vi "Double Motor Init.vi"(0 "Motor In":T2={"Motor1"={"DeviceStatus"={"status"=FALSE, "code"=0, "source"=""}, "Type"=enum."PWM", "PWM"={"PWM Channel"=enum."Invalid", "DeadBand"={"Name"="", "maxPositivePwm"=0, "minPositivePwm"=0, "centerPwm"=0, "maxNegativePwm"=0, "minNegativePwm"=0, "angularRange"=0}}, "CAN"={"Device Number"=0, "Control Mode"=enum."Percent VBus", "Semaphore"=refnum, "Max Vout"=12.0, "TalonSRX Control Mode"=enum."Percent VBus"}, "Invert"=FALSE}, "Motor2"={"DeviceStatus"={"status"=FALSE, "code"=0, "source"=""}, "Type"=enum."PWM", "PWM"={"PWM Channel"=enum."Invalid", "DeadBand"={"Name"="", "maxPositivePwm"=0, "minPositivePwm"=0, "centerPwm"=0, "maxNegativePwm"=0, "minNegativePwm"=0, "angularRange"=0}}, "CAN"={"Device Number"=0, "Control Mode"=enum."Percent VBus", "Semaphore"=refnum, "Max Vout"=12.0, "TalonSRX Control Mode"=enum."Percent VBus"}, "Invert"=FALSE}, "Last Motor Power"=0.0}, 1 "PWM Channel":T1, 5 "CAN Id":u8, 7 "Use Can":bool, 9 "Invert (default false)":bool, 11 "error in":errorcluster, 12 "PWM Channel 2":T1) -> (4 "Motor Out":T2={"Motor1"={"DeviceStatus"={"status"=FALSE, "code"=0, "source"=""}, "Type"=enum."PWM", "PWM"={"PWM Channel"=enum."Invalid", "DeadBand"={"Name"="", "maxPositivePwm"=0, "minPositivePwm"=0, "centerPwm"=0, "maxNegativePwm"=0, "minNegativePwm"=0, "angularRange"=0}}, "CAN"={"Device Number"=0, "Control Mode"=enum."Percent VBus", "Semaphore"=refnum, "Max Vout"=12.0, "TalonSRX Control Mode"=enum."Percent VBus"}, "Invert"=FALSE}, "Motor2"={"DeviceStatus"={"status"=FALSE, "code"=0, "source"=""}, "Type"=enum."PWM", "PWM"={"PWM Channel"=enum."Invalid", "DeadBand"={"Name"="", "maxPositivePwm"=0, "minPositivePwm"=0, "centerPwm"=0, "maxNegativePwm"=0, "minNegativePwm"=0, "angularRange"=0}}, "CAN"={"Device Number"=0, "Control Mode"=enum."Percent VBus", "Semaphore"=refnum, "Max Vout"=12.0, "TalonSRX Control Mode"=enum."Percent VBus"}, "Invert"=FALSE}, "Last Motor Power"=0.0}, 15 "error out":errorcluster)   [LabVIEW 2015]
uses:
  2 Motor Typedef.ctl
  <vilib>/Rock Robotics/WPI/MotorControl/WPI_MotorControlDeviceRef.ctl
  <vilib>/Rock Robotics/WPI/MotorControl/WPI_MotorControlType.ctl
  <vilib>/Rock Robotics/SystemInterfaces/DIO/FPGA_DIOPWMChannel.ctl
  <vilib>/Rock Robotics/WPI/PWM/WPI_PWMDeadband.ctl
  <vilib>/Rock Robotics/WPI/CAN/Jaguar/SubVIs/WPI_CANJaguar_ControlMode.ctl
  <vilib>/Rock Robotics/WPI/CAN/TalonSRX/WPI_CANTalonSRX_APIControlMode.ctl
  <vilib>/Rock Robotics/WPI/MotorControl/WPI_MotorControlOpenCANTalonSRX.vi
  <vilib>/Rock Robotics/WPI/MotorControl/WPI_MotorControlOpen VictorSP.vi
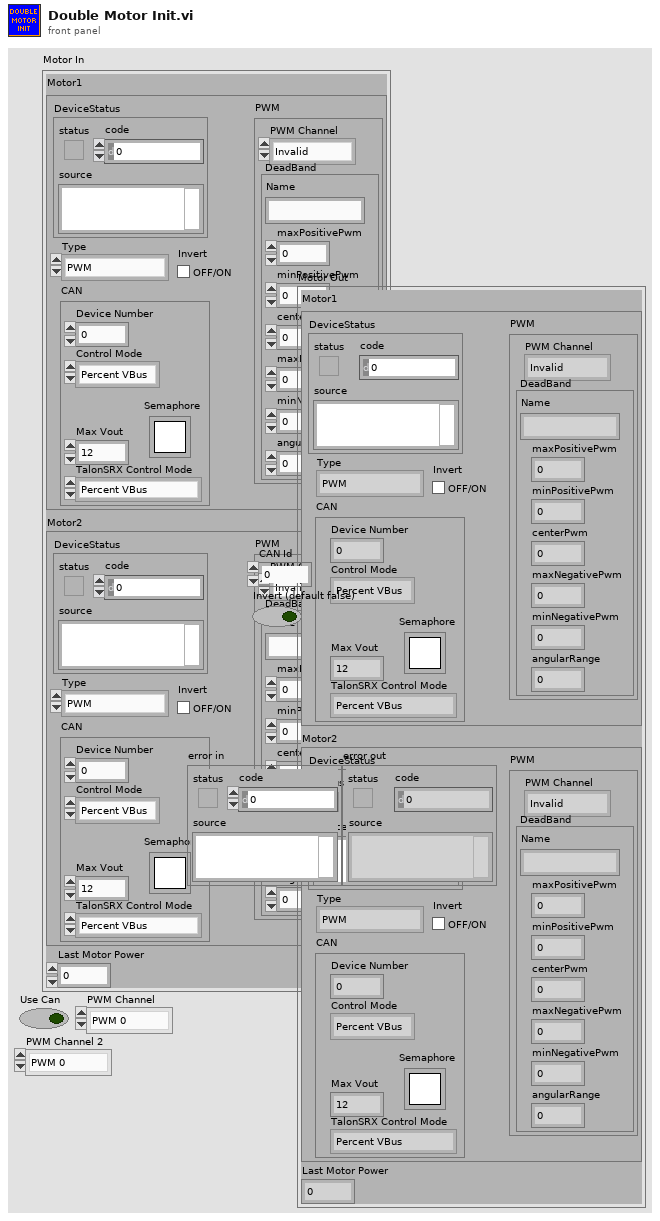
[diagram p1: front panel]
types:
  T1 = typedef "FPGA_DIOPWMChannel.ctl" = enum8{"PWM 0", "PWM 1", "PWM 2", "PWM 3", "PWM 4", "PWM 5", "PWM 6", "PWM 7", "PWM 8", "PWM 9", "PWM MXP 0", "PWM MXP 1", "PWM MXP 2", "PWM MXP 3", "PWM MXP 4", "PWM MXP 5", "PWM MXP 6", "PWM MXP 7", "PWM MXP 8", "PWM MXP 9", "Invalid"}
  T2 = typedef "2 Motor Typedef.ctl" = cluster{"Motor1":T3, "Motor2":T3, "Last Motor Power":dbl}
  T3 = typedef "WPI_MotorControlDeviceRef.ctl" = cluster{"DeviceStatus":errorcluster, "Type":T4, "PWM":cluster{"PWM Channel":T1, "DeadBand":T5}, "CAN":cluster{"Device Number":u8, "Control Mode":T6, "Semaphore":T7, "Max Vout":dbl, "TalonSRX Control Mode":T8}, "Invert":bool}
  T4 = typedef "WPI_MotorControlType.ctl" = enum16{"PWM", "CAN", "CANTalonSRX"}
  T5 = typedef "WPI_PWMDeadband.ctl" = cluster{"Name":string, "maxPositivePwm":i32, "minPositivePwm":i32, "centerPwm":i32, "maxNegativePwm":i32, "minNegativePwm":i32, "angularRange":u16}
  T6 = typedef "WPI_CANJaguar_ControlMode.ctl" = enum8{"Percent VBus", "Current", "Speed", "Position", "Voltage"}
  T7 = typedef "Semaphore RefNum" = refnum<k1>
  T8 = typedef "WPI_CANTalonSRX_APIControlMode.ctl" = enum8{"Percent VBus", "Speed", "Position", "Slave", "Unchanged / Invalid", "Voltage Compensation", "Current", "Motion Profile"}
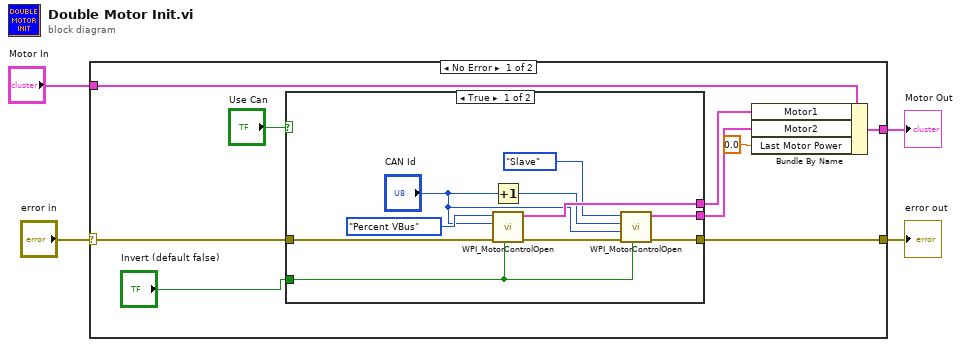
[diagram p0: block diagram]
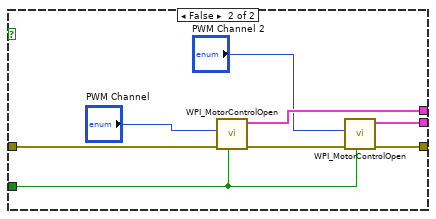
[diagram p2: hidden frame]
diagram:
  n1 = case shown="No Error" "error in" {
    selector: "error in" -> [w9 w32]
    tunnel: "Motor In" -> [w12 w33]
    tunnel: [w11 w33] -> w3
    tunnel: [w8 w32] -> w1
    frame No Error {
      n2 = case shown="True" "Use Can" {
        tunnel: [w23 w31] -> w13
        tunnel: [w17 w29] -> w10
        tunnel: w9 -> [w16 w28]
        tunnel: [w15 w27] -> w8
        tunnel: "Invert (default false)" -> [w14 w24]
        frame True {
          n3 = Increment(x="CAN Id") -> (x+1=w21:u8)
          n4 = call-poly <vilib>:"WPI_MotorControlOpen.vi"("Invert"=w14, "error in (no error)"=w16, "Device Number"="CAN Id", "Control Mode"=WPI_CANTalonSRX_APIControlMode."Percent VBus") -> ("error out"=w18:errorcluster, "MotorControlDeviceRef"=w23:T3)  [unwired: 6 in]
          n5 = call-poly <vilib>:"WPI_MotorControlOpen.vi"("Invert"=w14, "error in (no error)"=w18, "Master Device Number"="CAN Id", "Device Number"=w21, "Control Mode"=WPI_CANTalonSRX_APIControlMode."Slave") -> ("error out"=w15:errorcluster, "MotorControlDeviceRef"=w17:T3)  [unwired: 5 in]
        }
        frame False {
          n6 = call-poly <vilib>:"WPI_MotorControlOpen.vi"("Invert"=w24, "error in (no error)"=w28, "PWM Channel"="PWM Channel") -> ("error out"=w30:errorcluster, "MotorControlDeviceRef"=w31:T3)  [unwired: 7 in]
          n7 = call-poly <vilib>:"WPI_MotorControlOpen.vi"("Invert"=w24, "error in (no error)"=w30, "PWM Channel"="PWM Channel 2") -> ("error out"=w27:errorcluster, "MotorControlDeviceRef"=w29:T3)  [unwired: 7 in]
        }
      }
      n8 = Bundle By Name(cluster=w12, "Motor1"=w13, "Motor2"=w10, "Last Motor Power"=0.0) -> (w11:T2)
    }
    frame Error {
    }
  }
  "Motor Out" <- w3
  "error out" <- w1
